vi "Close.vi"(8 "error in (no error)":errorcluster, 11 "MKS MF1 in":refnum<class "PL MKS MF1 USB.lvclass">) -> (0 "error out":errorcluster)   [LabVIEW 2015, in "PL MKS MF1 USB.lvclass"]
doc: "Closes connection to device."
uses:
  PL MKS MF1 USB.lvclass
  PL MKS MF1 USB.lvclass/PL MKS MF1 USB.ctl
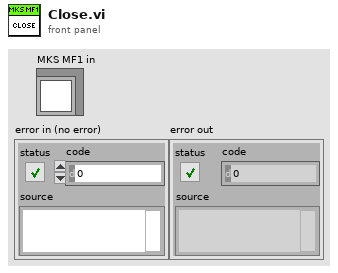
[diagram p1: front panel]
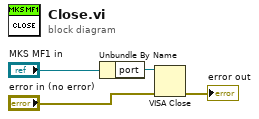
[diagram p0: block diagram]
diagram:
  n1 = Unbundle By Name("MKS MF1 in") -> ("port"=w3:refnum<visa-resource-name>)
  n2 = VISA Close(VISA resource name=w3, error in (no error)="error in (no error)") -> (error out=→"error out":errorcluster)
